vi "start.vi"   [LabVIEW 2017]
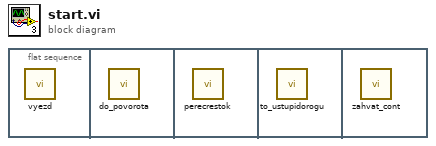
[diagram p0: block diagram]
diagram:
  n1 = flat-sequence {
    frame #0 {
      n2 = call "vyezd.vi"() -> ()  [unwired: 12 in]
    }
    frame #1 {
      n3 = call "do_povorota.vi"() -> ()  [unwired: 12 in]
    }
    frame #2 {
      n4 = call "perecrestok.vi"() -> ()  [unwired: 12 in]
    }
    frame #3 {
      n5 = call "to_ustupidorogu.vi"() -> ()  [unwired: 12 in]
    }
    frame #4 {
      n6 = call "zahvat_cont.vi"() -> ()  [unwired: 12 in]
    }
  }
